vi "Tree Delete Pulse.vi"(8 "error in (no error)":errorcluster, 10 "Shot":i32, 11 "Tree DVR in":refnum<data-value>) -> (0 "error out":errorcluster, 3 "Tree DVR out":refnum<data-value>)   [LabVIEW 2012, in "MDSplus.lvlib"]
doc: "Delete a pulse file."
uses:
  <vilib>/MDSplus/Library/MDSplus.lvlib
  <vilib>/MDSplus/Classes/Tree_Class/Tree.lvclass
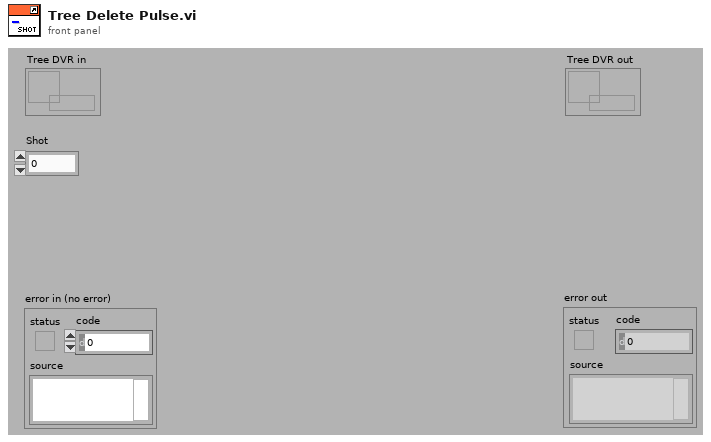
[diagram p1: front panel]
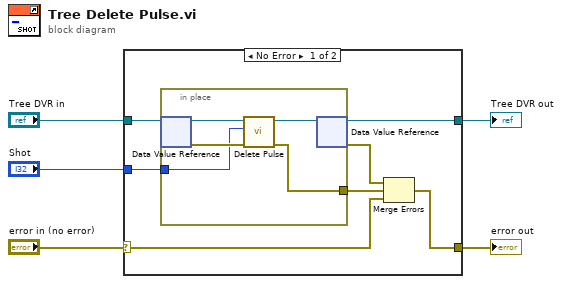
[diagram p0: block diagram]
diagram:
  n1 = case shown="No Error" "error in (no error)" {
    selector: "error in (no error)" -> [w11 w19]
    tunnel: "Tree DVR in" -> [w12 w18]
    tunnel: [w10 w19] -> w5
    tunnel: [w9 w18] -> w2
    tunnel: "Shot" -> [w8 _]
    frame No Error {
      n2 = in-place {
        in-place-border: [w13] -> w7
        in-place-border: w8 -> [w14]
        n3 = in-place-dvr #1(w12) -> (w17:refnum<class "Tree.lvclass">, w15:errorcluster)
        n4 = call-dynamic "Delete Pulse.vi"("error in (no error)"=w15, "Shot"=w14, "Tree in"=w17) -> ("error out"=w13:errorcluster, "Tree out"=w16:refnum<class "Tree.lvclass">)  [unwired: 7 in]
        n5 = in-place-dvr #1(w16) -> (w9:refnum<data-value>, w6:errorcluster)
      }
      n6 = Merge Errors(w6, w7, w11) -> (w10:errorcluster)
    }
    frame Error {
    }
  }
  "error out" <- w5
  "Tree DVR out" <- w2
